vi "Flock_Shared_Send Stop.vi"(8 "error in (no error)":errorcluster) -> (0 "error out":errorcluster)   [LabVIEW 2014, in "Flock_Shared_Messaging.lvlib" / "Flock_Shared_CentralProcessMessaging.lvlib"]
uses:
  Flock_Shared_CentralProcessMessaging.lvlib
  Flock_Shared_Messaging.lvlib
  FGV_Action.ctl
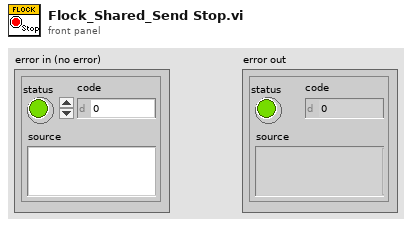
[diagram p1: front panel]
types:
  T1 = typedef "FGV_Action.ctl" = enum16{"Initalize Central", "Initialize Local", "Get", "Delete Local"}
  T2 = typedef "Flock_Shared_Messaging.lvlib/FGV_Queues.ctl" = cluster{"Local Queue in 2":T3, "Enum":T4}[]
  T3 = typedef "amc_Message Queue.ctl" = refnum<queue>
  T4 = typedef "Flock_Shared_Messaging.lvlib/ProcessList.ctl" = string
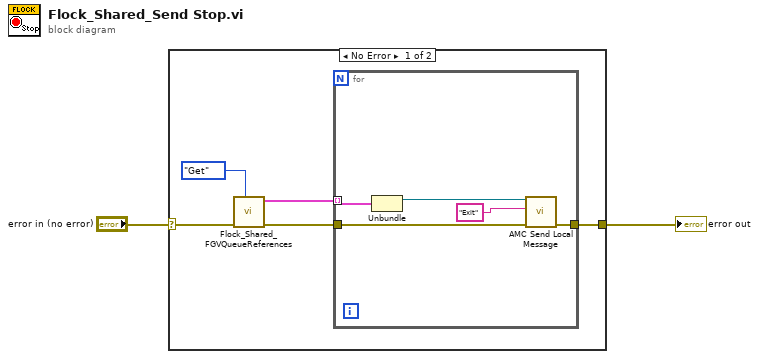
[diagram p0: block diagram]
diagram:
  n1 = case shown="No Error" "error in (no error)" {
    selector: "error in (no error)" -> [w3 w13]
    tunnel: [w7 w13] -> w2
    frame No Error {
      n2 = call "Flock_Shared_FGVQueueReferences.vi"("Action"=FGV_Action."Get", "error in (no error)"=w3) -> ("error out"=w6:errorcluster, "Array"=w5:T2)  [unwired: 7 in, 1 out]
      n3 = for {
        tunnel: [w12] -> w7
        tunnel: w6 -> [w8]
        tunnel: w5 -> [w10] mode=indexing
        n4 = Unbundle(w10) -> ("Local Queue in 2"=w9:T3)  [unwired: 1 out]
        n5 = call <vilib>:"AMC Send Local Message.vi"("error in (no error)"=w8, "Message Name"="Exit", "Message Queue in"=w9) -> ("error out"=w12:errorcluster)  [unwired: 7 in, 1 out]
      }
    }
    frame Error {
    }
  }
  "error out" <- w2
